vi "updateDisplaySettings.vi"(0 "Camera in":refnum<class "Camera.lvclass">, 5 "data_format":T1(ring)=enum."Mono16", 11 "error in (no error)":errorcluster) -> (4 "Camera out":refnum<class "Camera.lvclass">, 15 "error out":errorcluster)   [LabVIEW 2019, in "Camera.lvclass"]
doc: "Retreive the rec handle.\nThis handle allows direct access to all underlying functions of the pco.recorder."
uses:
  Camera.lvclass
  pco.convert/Convert.lvlib
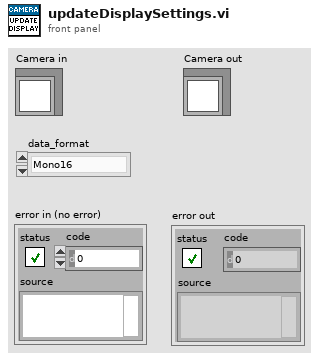
[diagram p1: front panel]
types:
  T1 = enum16{"Undefined", "Mono8", "Mono16", "BGRA8", "RGBA8", "BGRA16", "RGBA16", "CompressedMono8"}
  T2 = map{enum16{"Undefined", "Mono8", "Mono16", "BGRA8", "RGBA8", "BGRA16", "RGBA16", "CompressedMono8"}, u64}
  T3 = map{enum16{"Undefined", "Mono8", "Mono16", "BGRA8", "RGBA8", "BGRA16", "RGBA16", "CompressedMono8"}, cluster{"sharpen":bool, "adaptive_sharpen":bool, "flip_vertical":bool, "auto_minmax":bool, "min_limit":u16, "max_limit":u16, "gamma":dbl, "contrast":i32, "pco_debayer_algorithm":bool, "color_temperature":i32, "color_saturation":i32, "color_vibrance":i32, "color_tint":i32, "lut_file":path}}
  T4 = cluster{"sharpen":bool, "adaptive_sharpen":bool, "flip_vertical":bool, "auto_minmax":bool, "min_limit":u16, "max_limit":u16, "gamma":dbl, "contrast":i32, "pco_debayer_algorithm":bool, "color_temperature":i32, "color_saturation":i32, "color_vibrance":i32, "color_tint":i32, "lut_file":path}
  T5 = cluster{"wScale_minmax":u16, "iScale_maxmax":i32, "iScale_min":i32, "iScale_max":i32, "iColor_temp":i32, "iColor_tint":i32, "iColor_saturation":i32, "iColor_vibrance":i32, "iContrast":i32, "iGamma":i32, "iSRGB":i32, "pHistogramData":u64, "dwProcessingFlags":u32, "wProzValue4Min":u16, "wProzValue4Max":u16}
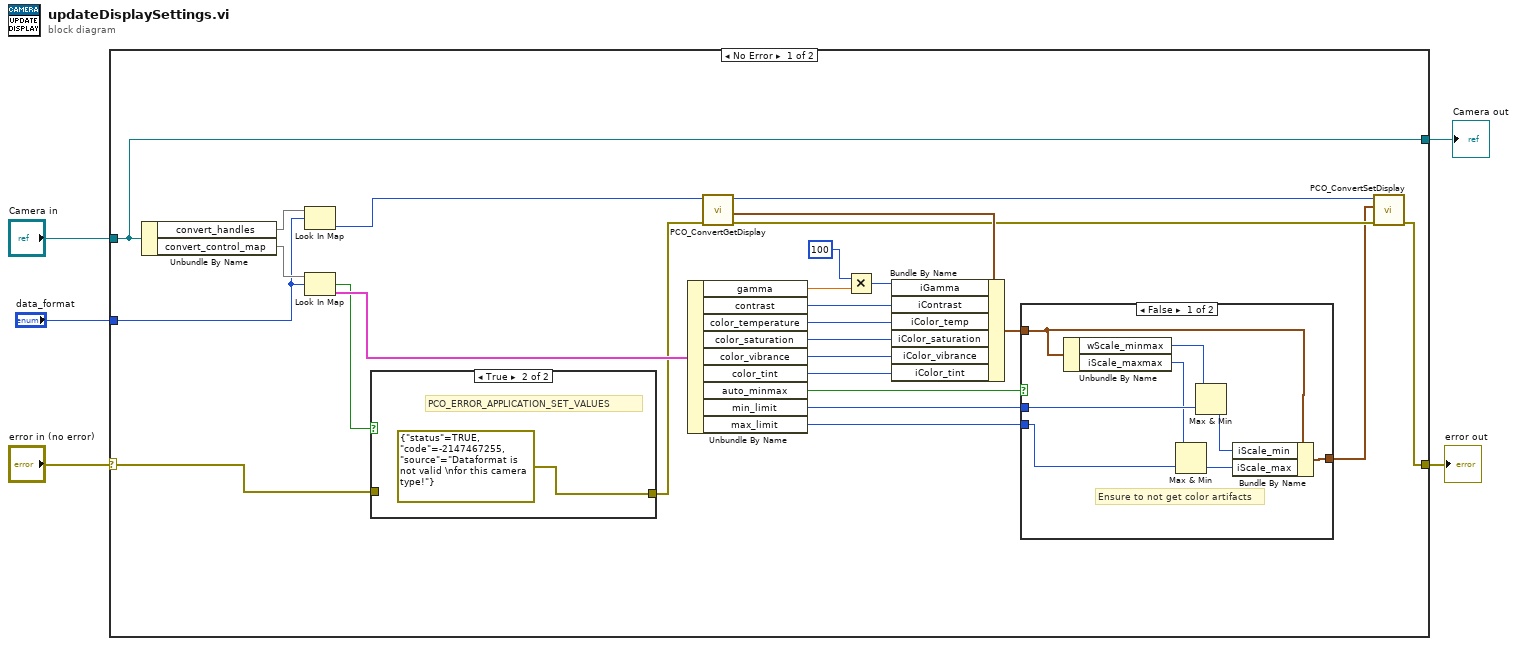
[diagram p0: block diagram]
diagram:
  n1 = case shown="No Error" "error in (no error)" {
    selector: "error in (no error)" -> [w21 w44]
    tunnel: [w16 w44] -> w3
    tunnel: [w15 w43] -> w4
    tunnel: "Camera in" -> [w15 w43]
    tunnel: "data_format" -> [w24 _]
    frame No Error {
      n2 = Unbundle By Name(w15) -> ("convert_handles"=w23:T2, "convert_control_map"=w25:T3)
      n3 = Look In Map(map=w23, key=w24) -> (value=w20:u64)  [unwired: 1 in, 1 out]
      n4 = Look In Map(map=w25, key=w24) -> (key not found?=w22:bool, value=w29:T4)  [unwired: 1 in]
      n5 = case shown="True" w22 {
        tunnel: w21 -> [w41 _]
        tunnel: [w41 errorcluster {"status"=TRUE, "code"=-2147467255, "source"="Dataformat is not valid \nfor this camera type!"} ("error IO")] -> w19
        frame False {
        }
        frame True {
          # "PCO_ERROR_APPLICATION_SET_VALUES"
        }
      }
      n6 = Unbundle By Name(w29) -> ("gamma"=w26:dbl, "contrast"=w14:i32, "color_temperature"=w13:i32, "color_saturation"=w12:i32, "color_vibrance"=w11:i32, "color_tint"=w10:i32, "auto_minmax"=w9:bool, "min_limit"=w8:u16, "max_limit"=w7:u16)
      n7 = call "PCO_ConvertGetDisplay.vi"("error in (no error)"=w19, "ph"=w20) -> ("error out"=w30:errorcluster, "strDisplay"=w31:T5, "ph out"=w17:u64)  [unwired: 6 in, 1 out]
      n8 = Multiply(x=100, y=w26) -> (x*y=w28:i32)
      n9 = Bundle By Name(cluster=w31, "iGamma"=w28, "iContrast"=w14, "iColor_temp"=w13, "iColor_saturation"=w12, "iColor_vibrance"=w11, "iColor_tint"=w10) -> (w6:T5)
      n10 = case shown="False" w9 {
        tunnel: w8 -> [w36 _]
        tunnel: w7 -> [w33 _]
        tunnel: [w39 w40] -> w18
        tunnel: w6 -> [w38 w40]
        frame False {
          # "Ensure to not get color artifacts"
          n11 = Unbundle By Name(w38) -> ("wScale_minmax"=w37:u16, "iScale_maxmax"=w34:i32)
          n12 = Max & Min(x=w34, y=w33) -> (min(x,y)=w32:i32)  [unwired: 1 out]
          n13 = Max & Min(x=w37, y=w36) -> (min(x,y)=w35:u16)  [unwired: 1 out]
          n14 = Bundle By Name(cluster=w38, "iScale_min"=w35, "iScale_max"=w32) -> (w39:T5)
        }
        frame True {
        }
      }
      n15 = call "PCO_ConvertSetDisplay.vi"("error in (no error)"=w30, "strDisplay"=w18, "ph"=w17) -> ("error out"=w16:errorcluster)  [unwired: 6 in, 2 out]
    }
    frame Error {
    }
  }
  "error out" <- w3
  "Camera out" <- w4
